vi "Build-Create Installer.vi"(0 "project in":refnum<vi>, 5 "iss name":string, 7 "version":string, 9 "slide in":refnum<vi>, 11 "error in (no error)":errorcluster) -> (15 "error out":errorcluster)   [LabVIEW 2020]
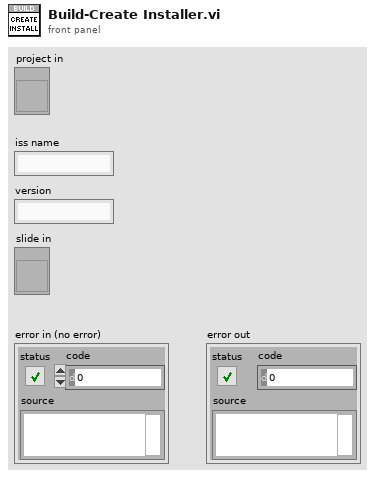
[diagram p1: front panel]
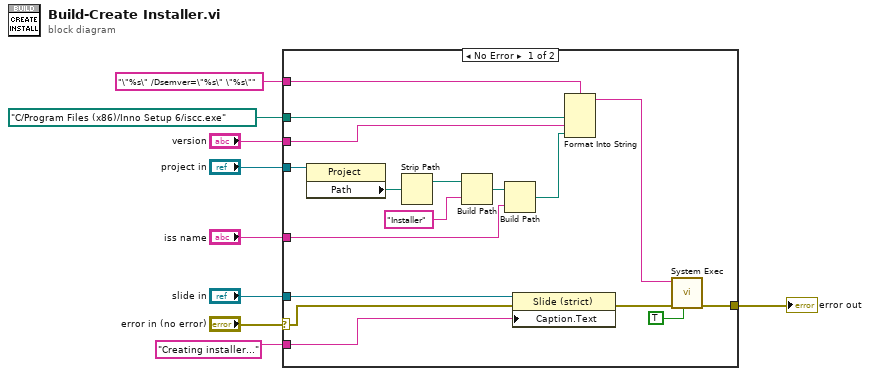
[diagram p0: block diagram]
diagram:
  n1 = case shown="No Error" "error in (no error)" {
    selector: "error in (no error)" -> [w20 w27]
    tunnel: [w26 w27] -> w6
    tunnel: "iss name" -> [w14 _]
    tunnel: "version" -> [w23 _]
    tunnel: path "C:/Program Files (x86)/Inno Setup 6/iscc.exe" -> [w22 _]
    tunnel: "\"%s\" /Dsemver=\"%s\" \"%s\"" ("command line") -> [w21 _]
    tunnel: "slide in" -> [w19 _]
    tunnel: "Creating installer..." ("Caption.Text") -> [w18 _]
    tunnel: "project in" -> [w16 _]
    frame No Error {
      n2 = property class="Project"(reference=w16) -> ("Path"=w11:path)  [unwired: 1 in, 2 out]
      n3 = Strip Path(path=w11) -> (stripped path=w10:path)  [unwired: 1 out]
      n4 = Build Path(base path=w10, name or relative path="Installer" ("Caption.Text")) -> (appended path=w15:path)
      n5 = Build Path(base path=w15, name or relative path=w14) -> (appended path=w13:path)
      n6 = property class="Slide (strict)"(reference=w19, error in=w20, "Caption.Text"=w18) -> (error out=w17:errorcluster)  [unwired: 1 out]
      n7 = Format Into String(format string=w21, w22, w23, w13) -> (resulting string=w25:string)  [unwired: 2 in, 1 out]
      n8 = call <vilib>:"System Exec.vi"("run minimized? (F)"=TRUE, "error in (no error)"=w17, "command line"=w25) -> ("error out"=w26:errorcluster)  [unwired: 5 in, 3 out]
    }
    frame Error {
    }
  }
  "error out" <- w6
